vi "TestReport.vi"() -> ()   [LabVIEW 2015]
uses:
  CustomControl/Report Info.ctl
  CustomControl/ReportTitle.ctl
panel:
  in  "Report":T1={"Title"={"订单数量"="12", "订单号"="1111", "生产代码"="2222", "日期"="12", "开始时间"="34", "结束时间"="56", "测试数量"="20", "预载荷时间"=2700, "载荷时间"=600, "检验员"="yao", "MLFB"="3RV6011-0AA10", "电流范围"="0.11-0.16", "起动时间"="", "快速时间范围"=""}, "uL"={"KTU"=["1.05", "1.2", "1.3", "1.4"], "Testing temp"=["21", "22", "23", "24"], "consTime"=200, "KG"=0.15, "Tripped Time"=[2500, 2600, 2700, 2800, 2900, 3000, 3100, 3200, 3300, 3400, 3500, 3600, 3700, 3800, 3900, 4000, 4100, 4200, 4300, 4400], "test?"=TRUE, "KGR"=[]}, "IL"={"KTU"=[], "Testing temp"=[], "consTime"=0, "KG"=0.0, "Tripped Time"=[], "test?"=FALSE, "KGR"=[]}, "Voltage"=[1.0, 2.0, 3.0, 4.0, 5.0, 6.0, 7.0, 8.0, 9.0, 10.0, 11.0, 12.0, 13.0, 14.0, 15.0, 16.0, 17.0, 18.0, 19.0, 20.0], "preLoad"=0, "Load"=0, "Total"=0, "JustCode"=[]}
  in  "Backup path":path=path "D:/3RV Software/CurrentTest2.xlsx"
  in  "Report path":path=path "D:/3RV Software/CurrentTest.xlsx"
  in  "template (empty)":path=path "D:/3RV Software/Source Code/Config/断路器极限电流试验报告.xlsx"
  out "error out":errorcluster
  out "Slide":u8(slide) scale=0.0..20.0
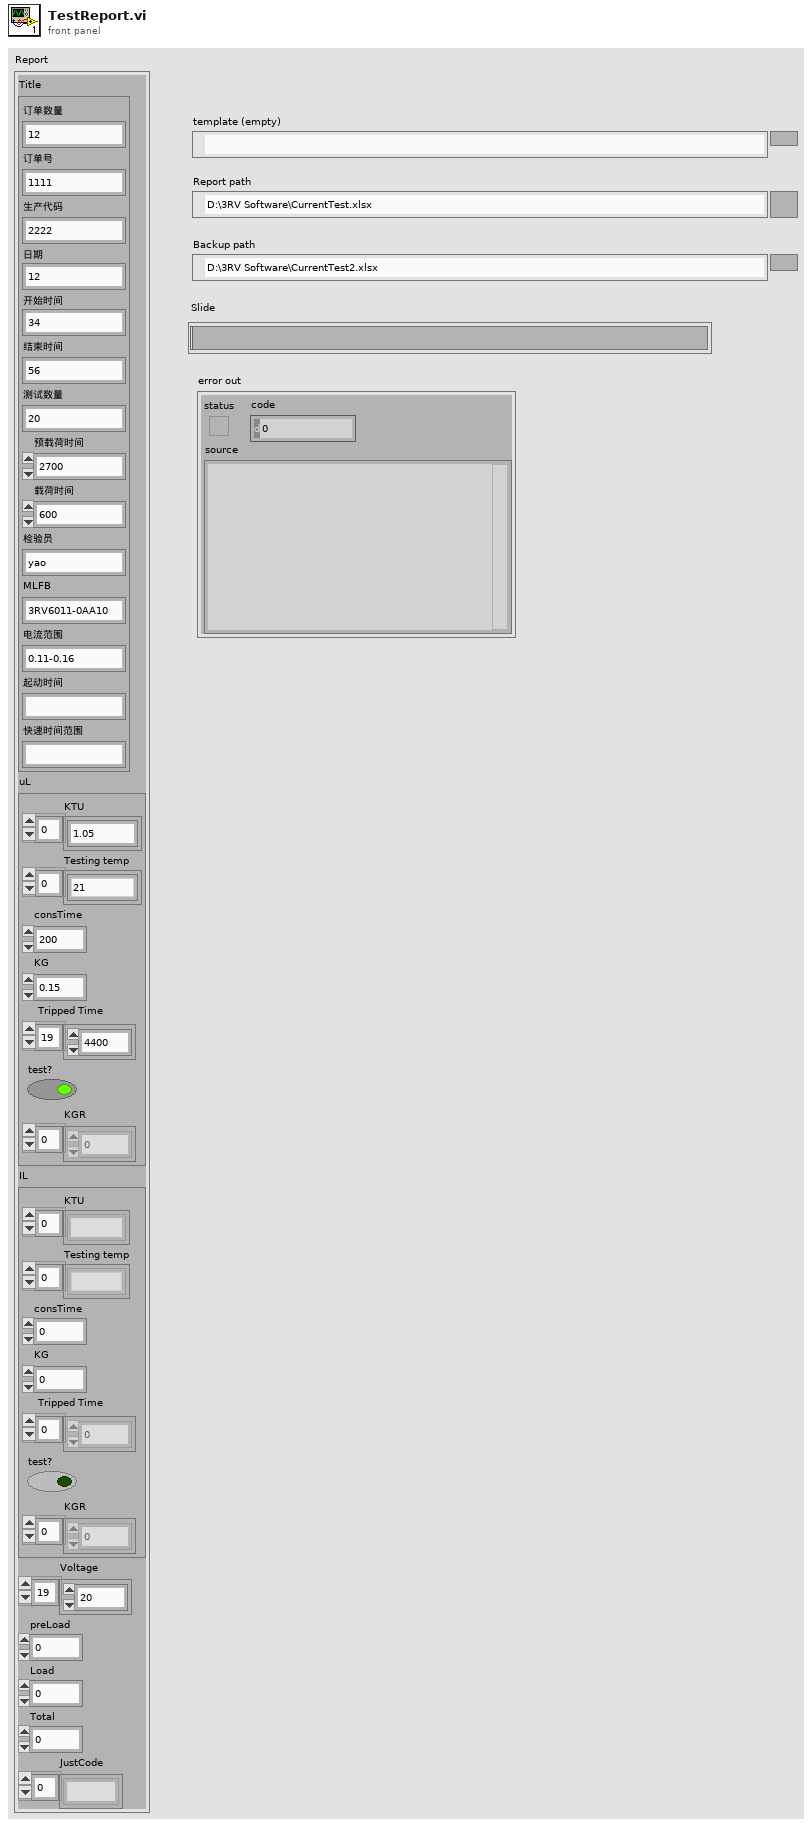
[diagram p1: front panel]
types:
  T1 = typedef "Report Info.ctl" = cluster{"Title":T2, "uL":cluster{"KTU":string[], "Testing temp":string[], "consTime":i32, "KG":dbl, "Tripped Time":i32[], "test?":bool, "KGR":dbl[]}, "IL":cluster{"KTU":string[], "Testing temp":string[], "consTime":i32, "KG":dbl, "Tripped Time":i32[], "test?":bool, "KGR":dbl[]}, "Voltage":dbl[], "preLoad":i32, "Load":i32, "Total":i32, "JustCode":string[]}
  T2 = typedef "ReportTitle.ctl" = cluster{"订单数量":string, "订单号":string, "生产代码":string, "日期":string, "开始时间":string, "结束时间":string, "测试数量":string, "预载荷时间":i32, "载荷时间":i32, "检验员":string, "MLFB":string, "电流范围":string, "起动时间":string, "快速时间范围":string}
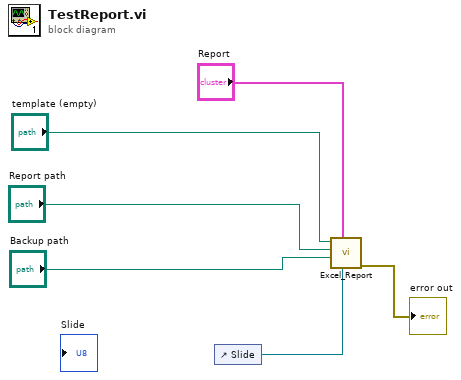
[diagram p0: block diagram]
diagram:
  n1 = control-ref of="Slide"() -> (w1:refnum<vi>)
  n2 = call "Excel_Report.vi"("Process"=w1, "Report"="Report", "Backup path"="Backup path", "Report path"="Report path", "template (empty)"="template (empty)") -> ("error out"=→"error out":errorcluster)  [unwired: 5 in, 1 out]
